vi "get_attribute.vi"(8 "error in (no error)":errorcluster, 11 "ClassA in":refnum<class "ClassA.lvclass">) -> (0 "error out":errorcluster, 2 "ClassB.lvclass":refnum<class "ClassB.lvclass">, 3 "ClassA out":refnum<class "ClassA.lvclass">)   [LabVIEW 2010, in "ClassA.lvclass"]
uses:
  ClassA.lvclass
  ClassB/ClassB.lvclass
  ClassA.lvclass/ClassA.ctl
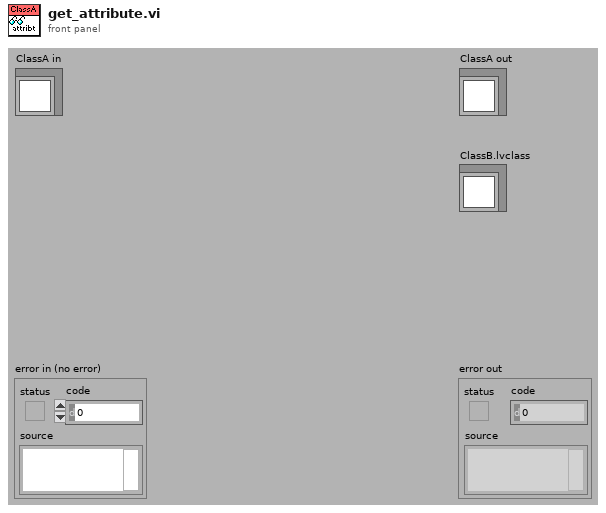
[diagram p1: front panel]
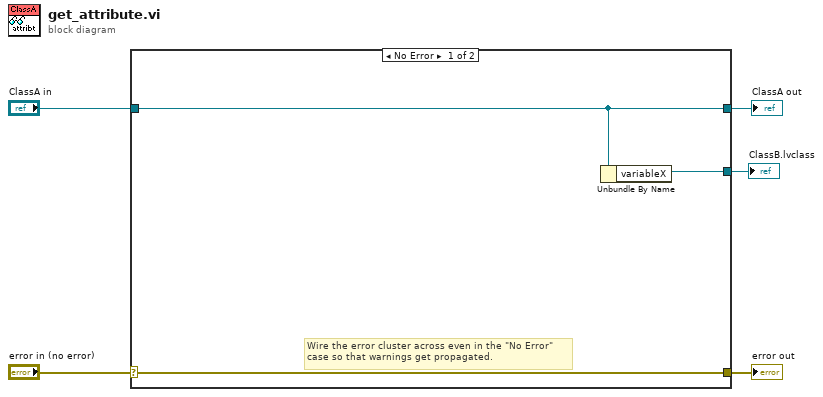
[diagram p0: block diagram]
diagram:
  n1 = case shown="No Error" "error in (no error)" {
    selector: "error in (no error)" -> [w8 w10]
    tunnel: [w8 w10] -> w4
    tunnel: [w6 w9] -> w2
    tunnel: "ClassA in" -> [w6 w9]
    tunnel: [w7 _] -> w1
    frame No Error {
      # "Wire the error cluster across even in the \"No Error\"\ncase so that warnings get propagated."
      n2 = Unbundle By Name(w6) -> ("variableX"=w7:refnum<class "ClassB.lvclass">)
    }
    frame Error {
    }
  }
  "error out" <- w4
  "ClassA out" <- w2
  "ClassB.lvclass" <- w1
